vi "set_controls_enabled_state.vi"(8 "error in (no error)":errorcluster, 9 "status":T1(ring), 10 "control references":refnum<vi>[](array[refnum]), 11 "ImagingModeDL090130Frame in":refnum<class "ImagingModeDL090130Frame.lvclass">=refnum) -> (0 "error out":errorcluster, 3 "ImagingModeDL090130Frame out":refnum<class "ImagingModeDL090130Frame.lvclass">)   [LabVIEW 2010, in "ImagingModeDL090130Frame.lvclass"]
uses:
  ImagingModeDL090130Frame.lvclass
  ImagingModeDL090923Scaffold/ImagingModeDL090923Scaffold/ImagingModeDL090923Scaffold.lvclass
  main/labview_source/type_definitions/enumerations/run_mode_enum.ctl
  ImagingModeDL090130Frame.lvclass/ImagingModeDL090130Frame.ctl
  common/classes/GenericComponent/GenericComponent/class_data.vi
  common/classes/ErrorController/ErrorController/class_data.vi
  common/classes/ErrorController/ErrorController/ErrorController.lvclass
  common/classes/GenericComponent/GenericComponent/GenericComponent.lvclass
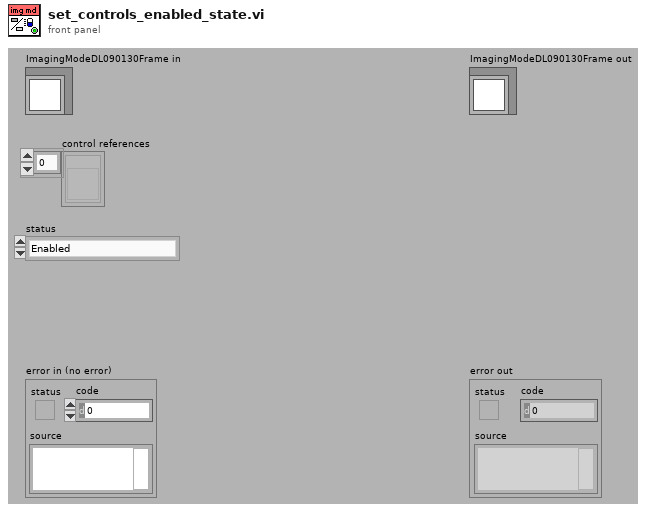
[diagram p1: front panel]
types:
  T1 = enum8{"Enabled", "Disabled", "Disabled and Grayed Out"}
  T2 = typedef "run_mode_enum.ctl" = enum16{"focus mode", "single sweep mode", "experiment mode"}
  T3 = typedef "ImagingModeDL090130Frame.lvclass/control_refs.ctl" = cluster{"resolution controls":cluster{"x pixels":refnum<vi>, "y pixels":refnum<vi>, "ratio x factor":refnum<vi>, "ratio y factor":refnum<vi>}, "speed controls":cluster{"pixel dwell time":refnum<vi>, "line scan time":refnum<vi>, "frame rate":refnum<vi>}, "number of frames controls":cluster{"# of frames":refnum<vi>, "duration":refnum<vi>, "# of repetitions":refnum<vi>}, "current value indicators":cluster{"frame #":refnum<vi>, "repetition #":refnum<vi>, "offset":refnum<vi>}, "step controls":cluster{"step size":refnum<vi>, "return to origin?":refnum<vi>, "translation mode":refnum<vi>, "XIntensityCompensation":refnum<vi>}, "settings":refnum<vi>, "defineButton":refnum<vi>, "settings enforced?":refnum<vi>}
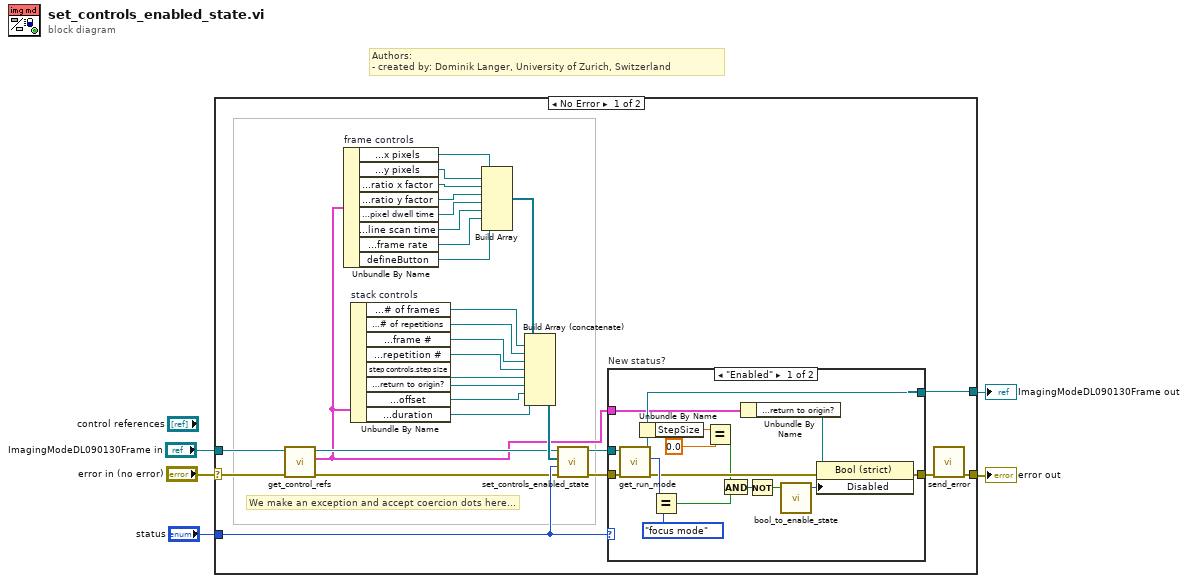
[diagram p0: block diagram]
diagram:
  # "Authors: \n- created by: Dominik Langer, University of Zurich, Switzerland"
  n1 = case shown="No Error" "error in (no error)" {
    selector: "error in (no error)" -> [w10 w54]
    tunnel: [w13 w54] -> w4
    tunnel: [w34 w53] -> w2
    tunnel: "ImagingModeDL090130Frame in" -> [w8 w53]
    tunnel: "status" -> [w16 _]
    frame No Error {
      # "We make an exception and accept coercion dots here..."
      n2 = call-dynamic "get_control_refs.vi"("error in (no error)"=w10, "ImagingModeDL090130Frame in"=w8) -> ("error out"=w9:errorcluster, "control refs"=w6:T3, "ImagingModeDL090130Frame out"=w7:refnum<class "ImagingModeDL090130Frame.lvclass">)  [unwired: 7 in]
      n3 = Unbundle By Name "frame controls"(w6) -> ("resolution controls.x pixels"=w22:refnum<vi>, "resolution controls.y pixels"=w21:refnum<vi>, "resolution controls.ratio x factor"=w24:refnum<vi>, "resolution controls.ratio y factor"=w25:refnum<vi>, "speed controls.pixel dwell time"=w19:refnum<vi>, "speed controls.line scan time"=w20:refnum<vi>, "speed controls.frame rate"=w23:refnum<vi>, "defineButton"=w11:refnum<vi>)
      n4 = Unbundle By Name "stack controls"(w6) -> ("number of frames controls.# of frames"=w33:refnum<vi>, "number of frames controls.# of repetitions"=w32:refnum<vi>, "current value indicators.frame #"=w31:refnum<vi>, "current value indicators.repetition #"=w30:refnum<vi>, "step controls.step size"=w28:refnum<vi>, "step controls.return to origin?"=w26:refnum<vi>, "current value indicators.offset"=w29:refnum<vi>, "number of frames controls.duration"=w27:refnum<vi>)
      n5 = Build Array(w22, w21, w24, w25, w19, w20, w23, w11) -> (w14:refnum<vi>[])
      n6 = Build Array (concatenate)(w14, w33, w32, w31, w30, w28, w26, w29, w27) -> (w15:refnum<vi>[])
      n7 = call-parent "set_controls_enabled_state.vi"("error in (no error)"=w9, "status"=w16, "control references"=w15, "GenericPlugin in"=w7) -> ("error out"=w18:errorcluster, "GenericPlugin out"=w17:refnum<class "ImagingModeDL090130Frame.lvclass">)  [unwired: 6 in]
      n8 = case "New status?" shown="\"Enabled\"" w16 {
        tunnel: w18 -> [w49 w52]
        tunnel: [w50 w52] -> w12
        tunnel: w17 -> [w48 w51]
        tunnel: [w47 w51] -> w34
        tunnel: w6 -> [w43 _]
        frame "Enabled" {
          n9 = call "get_run_mode.vi"("error in (no error)"=w49, "GenericPlugin in"=w48) -> ("error out"=w36:errorcluster, "run mode"=w46:T2, "GenericPlugin out"=w47:refnum<class "ImagingModeDL090130Frame.lvclass">)  [unwired: 5 in, 2 out]
          n10 = Unbundle By Name(w47) -> ("StepSize"=w38:dbl[unit])
          n11 = Equal?(x=w46, y=run_mode_enum."focus mode") -> (x = y?=w44:bool)
          n12 = Equal?(x=w38, y=dbl[unit] 0.0) -> (x = y?=w35:bool)
          n13 = And(x=w35, y=w44) -> (x .and. y?=w41:bool)
          n14 = Unbundle By Name(w43) -> ("step controls.return to origin?"=w42:refnum<vi>)
          n15 = Not(x=w41) -> (.not. x?=w40:bool)
          n16 = call "bool_to_enable_state.vi"("boolean in"=w40) -> ("enabled status out"=w39:T1)  [unwired: 4 in]
          n17 = property class="Bool (strict)"(reference=w42, error in=w36, "Disabled"=w39) -> (error out=w50:errorcluster)  [unwired: 1 out]
        }
        frame "Disabled", Default {
        }
      }
      n18 = call "send_error.vi"("error in (no error)"=w12) -> ("error out"=w13:errorcluster)  [unwired: 10 in]
    }
    frame Error {
    }
  }
  "error out" <- w4
  "ImagingModeDL090130Frame out" <- w2
